vi "BoundaryAndCorrection.vi"() -> ()   [LabVIEW 2017]
uses:
  <vilib>/express/express arith-compare/Formula/XNode/ExpressFormulaBlockNode.xnode
panel:
  out "Omega":dbl=0.011911070482791955
  in  "Zmax":dbl=280.0 format="%#_13g"
  in  "Zmin":dbl=-60.0 format="%#_13g"
  in  "Xmax":dbl=320.0 format="%#_13g"
  in  "Xmin":dbl=95.0 format="%#_13g"
  out "Z1":dbl=140.74534161490683 format="%#_13g"
  out "Y1":dbl=3.6641221374045756 format="%#_13g"
  out "X1":dbl=301.7391304347826 format="%#_13g"
  out "Within Bounds?":bool=TRUE
  out "C5":bool=TRUE
  out "C4":bool=TRUE
  out "C3":bool=TRUE
  out "C2":bool=TRUE
  out "C1":bool=TRUE
  in  "Epsilon":dbl=10.0 format="%#_13g"
  out "Z":dbl=34.64534161490684
  out "X":dbl=244.0613769629516
  in  "Beta":dbl=0.209 format="%#_13g"
  in  "Theta":dbl=0.126 format="%#_13g"
  in  "Phi":dbl=0.367 format="%#_13g"
  in  "R3":dbl=288.0 format="%#_13g"
  in  "Alpha":dbl=0.68 format="%#_13g"
  in  "R1":dbl=142.0 format="%#_13g"
  in  "R2":dbl=158.8 format="%#_13g"
  in  "Tz":dbl=106.1 format="%#_13g"
  in  "Tx":dbl=57.7 format="%#_13g"
  in  "Zo":dbl(slide)=140.74534161490683 scale=-70.0..320.0
  in  "Yo":dbl(slide)=3.6641221374045756 scale=-160.0..160.0
  in  "Xo":dbl(slide)=301.7391304347826 scale=65.0..380.0
  # "Given"
  # "Subject to Change"
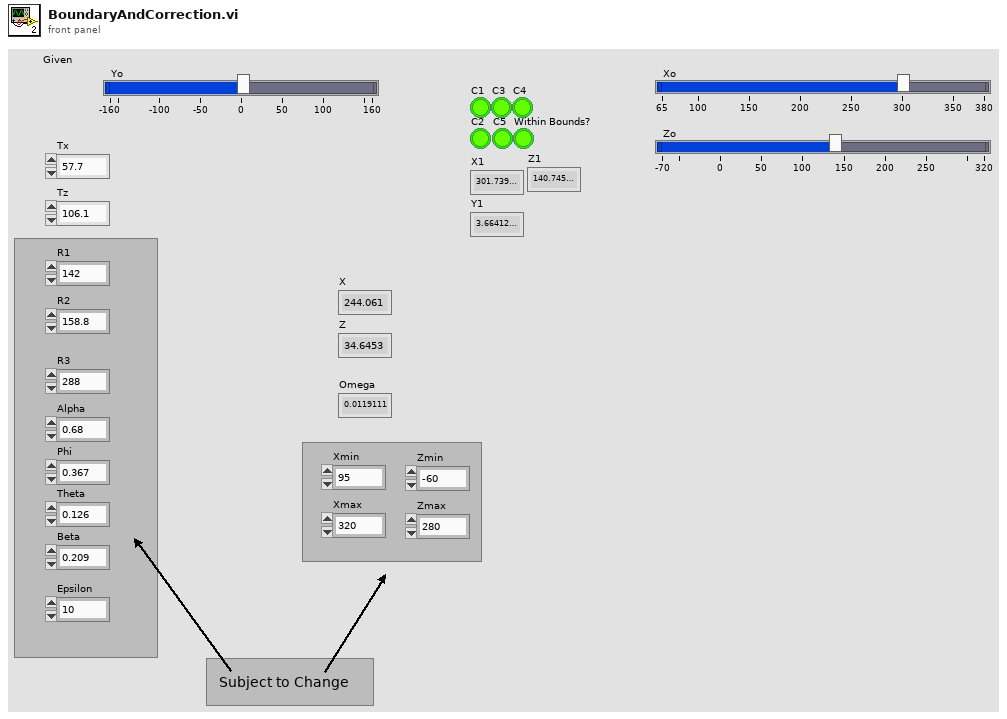
[diagram p1: front panel]
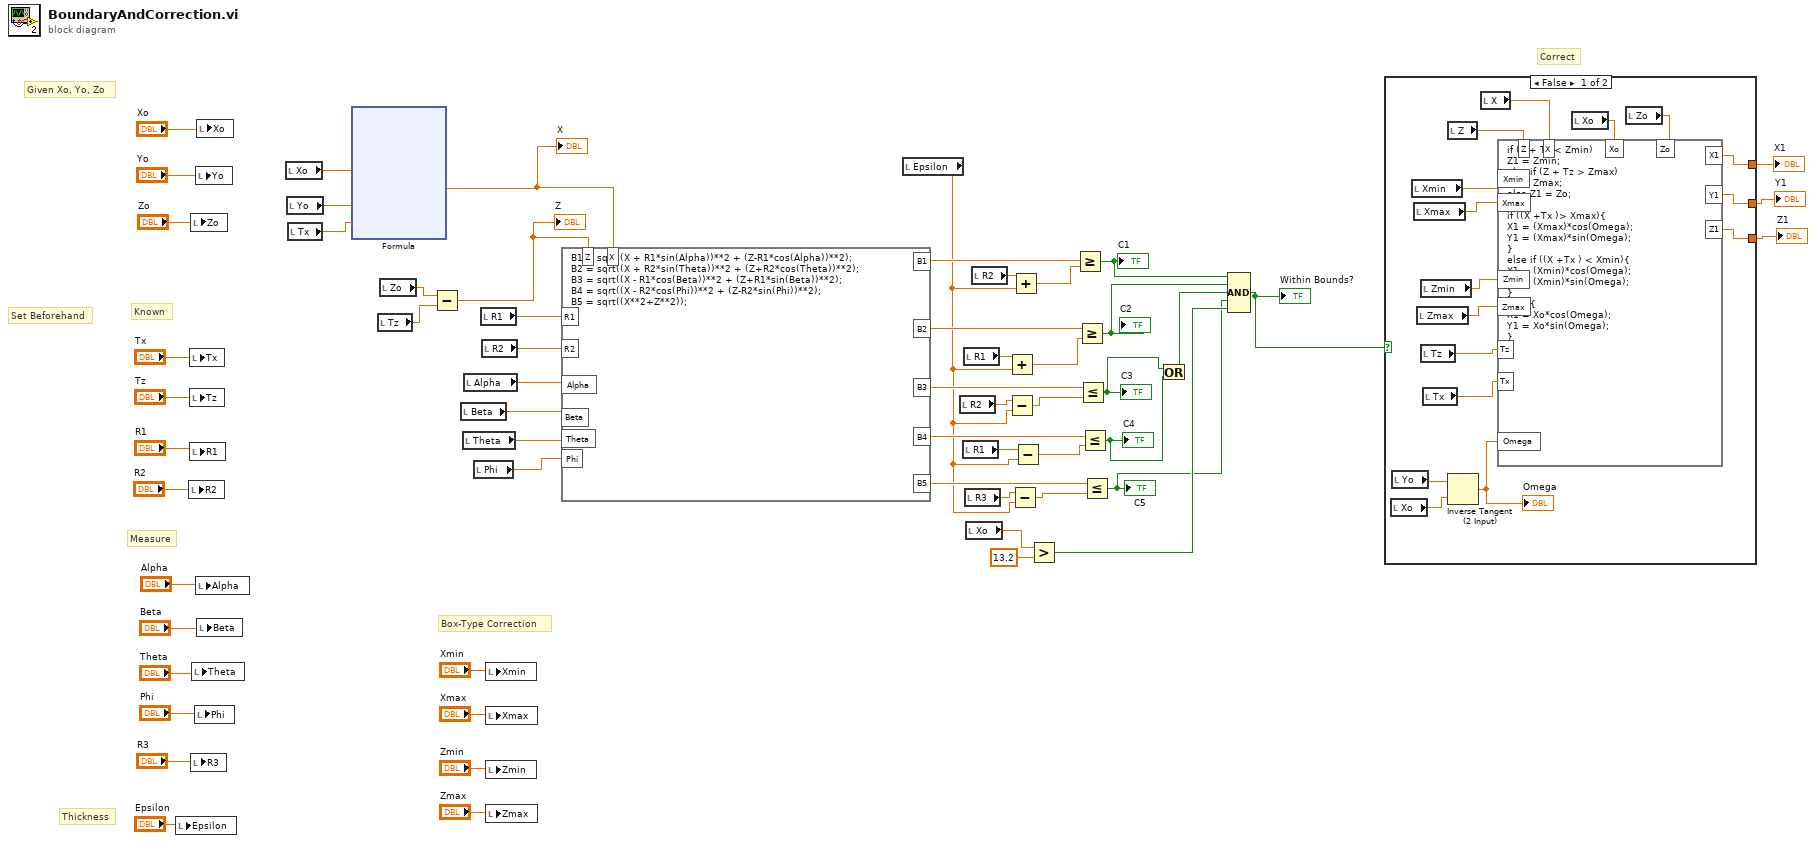
[diagram p0: block diagram]
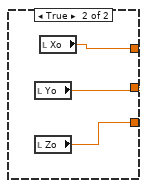
[diagram p2: hidden frame]
diagram:
  # "Box-Type Correction"
  # "Correct"
  # "Thickness"
  # "Known"
  # "Measure"
  # "Set Beforehand"
  # "Given Xo, Yo, Zo"
  n1 = local write "Epsilon"("Epsilon") -> ()
  n2 = local write "R2"("R2") -> ()
  n3 = local write "Tx"("Tx") -> ()
  n4 = local write "Tz"("Tz") -> ()
  n5 = local write "R1"("R1") -> ()
  n6 = local write "Zo"("Zo") -> ()
  n7 = local write "R3"("R3") -> ()
  n8 = local write "Theta"("Theta") -> ()
  n9 = local write "Phi"("Phi") -> ()
  n10 = local write "Yo"("Yo") -> ()
  n11 = local write "Alpha"("Alpha") -> ()
  n12 = local write "Xo"("Xo") -> ()
  n13 = local write "Beta"("Beta") -> ()
  n14 = local read "Xo"() -> (w47:dbl)
  n15 = local read "Yo"() -> (w46:dbl)
  n16 = local read "Tx"() -> (w45:dbl)
  n17 = xnode "Formula"("Xo"=w47, "Yo"=w46, "Tx"=w45) -> ("Result"=w39:dbl)  [unwired: 1 in, 1 out]
  "X" <- w39
  n18 = local read "Tz"() -> (w43:dbl)
  n19 = local read "Zo"() -> (w44:dbl)
  n20 = Subtract(x=w44, y=w43) -> (x-y=w38:dbl)
  "Z" <- w38
  n21 = local read "Beta"() -> (w36:dbl)
  n22 = local read "Theta"() -> (w35:dbl)
  n23 = local read "Alpha"() -> (w37:dbl)
  n24 = local read "Phi"() -> (w34:dbl)
  n25 = local read "R1"() -> (w41:dbl)
  n26 = local read "R2"() -> (w40:dbl)
  n27 = local write "Xmin"("Xmin") -> ()
  n28 = local write "Xmax"("Xmax") -> ()
  n29 = local write "Zmin"("Zmin") -> ()
  n30 = local write "Zmax"("Zmax") -> ()
  n31 = formula code="B1 = sqrt((X + R1*sin(Alpha))**2 + (Z-R1*cos(Alpha))**2);\nB2 = sqrt((X + R2*sin(Theta))**2 + (Z+R2*cos(Theta))**2);\nB3 = sqrt((X - R1*cos(Beta))**2 + (Z+R1*sin(Beta))**2);\nB4 = sqrt((X - R2*cos(Phi))**2 + (Z-R2*sin(Phi))**2);\nB5 = sqrt((X**2+Z**2));"("R1"=w41, "R2"=w40, "X"=w39, "Z"=w38, "Alpha"=w37, "Beta"=w36, "Theta"=w35, "Phi"=w34) -> ("B1"=w33:dbl, "B2"=w29:dbl, "B3"=w27:dbl, "B4"=w23:dbl, "B5"=w21:dbl)
  n32 = local read "Epsilon"() -> (w18:dbl)
  n33 = local read "R2"() -> (w26:dbl)
  n34 = local read "R1"() -> (w24:dbl)
  n35 = local read "R1"() -> (w30:dbl)
  n36 = local read "R3"() -> (w19:dbl)
  n37 = local read "Xo"() -> (w15:dbl)
  n38 = local read "R2"() -> (w32:dbl)
  n39 = Add(x=w30, y=w18) -> (x+y=w28:dbl)
  n40 = Subtract(x=w26, y=w18) -> (x-y=w25:dbl)
  n41 = Subtract(x=w19, y=w18) -> (x-y=w20:dbl)
  n42 = Add(x=w32, y=w18) -> (x+y=w31:dbl)
  n43 = Subtract(x=w24, y=w18) -> (x-y=w22:dbl)
  n44 = Greater?(x=w15, y=13.2) -> (0:w5:bool)
  n45 = Greater Or Equal?(x=w33, y=w31) -> (x >= y?=w17:bool)
  "C1" <- w17
  n46 = Greater Or Equal?(x=w29, y=w28) -> (x >= y?=w16:bool)
  "C2" <- w16
  n47 = Less Or Equal?(x=w27, y=w25) -> (x <= y?=w3:bool)
  "C3" <- w3
  n48 = Less Or Equal?(x=w23, y=w22) -> (x <= y?=w4:bool)
  "C4" <- w4
  n49 = Less Or Equal?(x=w21, y=w20) -> (x <= y?=w1:bool)
  "C5" <- w1
  n50 = Or(x=w3, y=w4) -> (x .or. y?=w2:bool)
  n51 = Compound Arithmetic op=AND(w17, w16, w2, w1, w5) -> (w13:bool)
  "Within Bounds?" <- w13
  n52 = case shown="False" w13 {
    tunnel: [w65 w78] -> w12
    tunnel: [w64 w77] -> w11
    tunnel: [w69 w76] -> w10
    frame False {
      n53 = local read "Xo"() -> (w68:dbl)
      n54 = local read "Yo"() -> (w67:dbl)
      n55 = local read "Xmin"() -> (w71:dbl)
      n56 = local read "Xmax"() -> (w70:dbl)
      n57 = local read "Zmax"() -> (w72:dbl)
      n58 = local read "Zmin"() -> (w73:dbl)
      n59 = local read "Tz"() -> (w63:dbl)
      n60 = local read "Tx"() -> (w62:dbl)
      n61 = local read "Z"() -> (w75:dbl)
      n62 = Inverse Tangent (2 Input)(1:w68, 2:w67) -> (0:w66:dbl)
      "Omega" <- w66
      n63 = local read "X"() -> (w74:dbl)
      n64 = local read "Xo"() -> (w61:dbl)
      n65 = local read "Zo"() -> (w60:dbl)
      n66 = formula code="if (Z + Tz < Zmin)\nZ1 = Zmin;\nelse if (Z + Tz > Zmax)\nZ1 = Zmax;\nelse Z1 = Zo;\n\nif ((X +Tx )> Xmax){\nX1 = (Xmax)*cos(Omega);\nY1 = (Xmax)*sin(Omega);\n}\nelse if ((X +Tx ) < Xmin){\nX1 = (Xmin)*cos(Omega);\nY1 = (Xmin)*sin(Omega);\n}\nelse {\nX1 = Xo*cos(Omega);\nY1 = Xo*sin(Omega);\n}"("X"=w74, "Z"=w75, "Zmin"=w73, "Zmax"=w72, "Xmin"=w71, "Xmax"=w70, "Omega"=w66, "Tz"=w63, "Tx"=w62, "Xo"=w61, "Zo"=w60) -> ("Z1"=w69:dbl, "X1"=w65:dbl, "Y1"=w64:dbl)
    }
    frame True {
      n67 = local read "Yo"() -> (w77:dbl)
      n68 = local read "Zo"() -> (w76:dbl)
      n69 = local read "Xo"() -> (w78:dbl)
    }
  }
  "X1" <- w12
  "Y1" <- w11
  "Z1" <- w10
